vi "Write Action.vi"(8 "error in (no error)":errorcluster, 10 "Action":T1, 11 "Background Loop Msg in":refnum<class "Background Loop Msg.lvclass">) -> (0 "error out":errorcluster, 3 "Background Loop Msg out":refnum<class "Background Loop Msg.lvclass">)   [LabVIEW 2021, in "Background Loop Msg.lvclass"]
uses:
  Background Loop Msg.lvclass
  Worker Actor/Background Loop Action.ctl
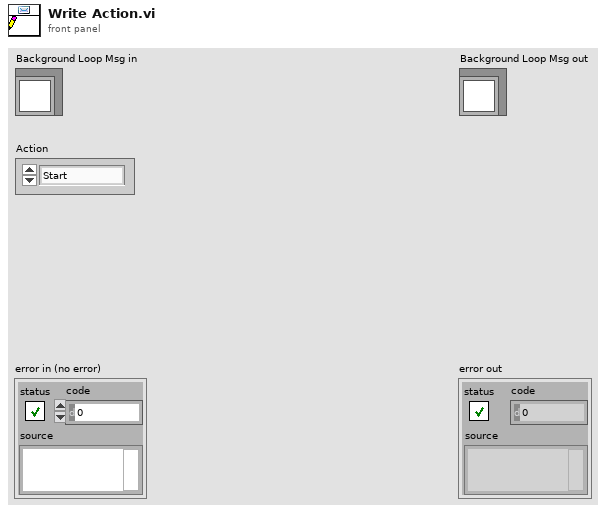
[diagram p1: front panel]
types:
  T1 = typedef "Background Loop Action.ctl" = enum16{"Start", "Continue", "Stop"}
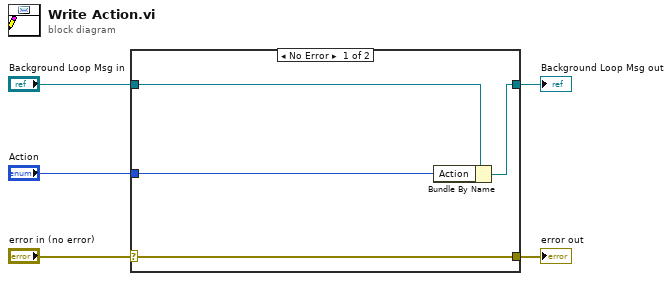
[diagram p0: block diagram]
diagram:
  n1 = case shown="No Error" "error in (no error)" {
    selector: "error in (no error)" -> [w9 w10]
    tunnel: [w9 w10] -> w4
    tunnel: [w7 w11] -> w2
    tunnel: "Background Loop Msg in" -> [w8 w11]
    tunnel: "Action" -> [w6 _]
    frame No Error {
      n2 = Bundle By Name(cluster=w8, "Action"=w6) -> (w7:refnum<class "Background Loop Msg.lvclass">)
    }
    frame Error {
    }
  }
  "error out" <- w4
  "Background Loop Msg out" <- w2
